vi "CalWAM-Prod(BETA).vi"(11 "error in (no error)":errorcluster) -> (4 "reference out":refnum<vi>, 15 "error out":errorcluster)   [LabVIEW 2018]
uses:
  <vilib>/Utility/file.llb/Write Delimited Spreadsheet (string).vi
  <vilib>/Utility/file.llb/Write Delimited Spreadsheet (DBL).vi
  Instruments/Keysight U2022 Power Sensor/Agilent U2000 Series/Agilent U2000 Series.lvlib
  Instruments/Agilent PSG MXG Series/Agilent PSG MXG Series.lvlib
panel:
  in  "gantry_Required(t)":bool=TRUE
  in  "Gantry":refnum<visa-resource-name>="COM5"
  in  "Path":u16(ring)=3 items=["INPUT", "FLATTEN", "OUTPUT"]
  out "IsPSA?(t)":bool
  out "SA_Offset":dbl=-100.433
  out "sg_flat_temp":path=path "C:/Users/ThomasWattson/AppData/Local/Temp/lvtemporary_990258.cal"
  out "in_cal_temp":path=path "C:/Users/ThomasWattson/AppData/Local/Temp/lvtemporary_29106.cal"
  out "out_cal_tmp":path=path "C:/Users/ThomasWattson/AppData/Local/Temp/lvtemporary_754512.cal"
  out "in_cal_file":path=path "C:/RageATE/Automated Tests/Tetra WAM/PRODUCTION/Test Benches/WAM_PROD_TEST-2/Calibration Files/WAM_PROD_TEST-2_INPUT_072523-1034.csv"
  out "date/time string":string="072523-1034"
  out "TestBench_ID":string="WAM_PROD_TEST-2"
  out "Cancel_@_Inst":bool
  in  "Tab Control":enum32{"CAL", "INST"}(tab)
  out "Switch_Present?(t)":bool=TRUE
  out "PM_Present?(t)":bool=TRUE
  out "VNA_Present?(t)":bool=TRUE
  out "MXG_Present?(t)":bool=TRUE
  out "MXA_Present?(t)":bool=TRUE
  in  "stop":bool
  out "Progress":u8(slide) caption="Input Cal 100% Complete" scale=0.0..100.0
  out "Status":string="Starting:  CalWAM-Prod(BETA).vi\rChecking Equipment..."
  out "Spec An":dbl[](array[numeric])=[11000.0, -100.433]
  out "Power Meter":dbl[](array[numeric])=[10000.0, -41.4955603]
  in  "USB Power Meter":refnum<visa-resource-name>="USB0::0x2A8D::0x7F18::MY58240013::INSTR"
  in  "VNA":refnum<visa-resource-name>="TCPIP0::169.254.70.180::inst0::INSTR"
  in  "SA":refnum<visa-resource-name>="TCPIP0::169.254.70.120::inst0::INSTR"
  in  "Sig Gen":refnum<visa-resource-name>="TCPIP0::169.254.70.100::inst0::INSTR"
  in  "PM_AVGs":i16=4
  in  "SA_AVGs":i16=8
  in  "Switch":refnum<visa-resource-name>="GPIB0::29::INSTR"
  in  "MXA_Required(t)":bool=TRUE
  in  "Preset_MXA(t)":bool=TRUE
  in  "Preset_MXG(t)":bool=TRUE
  in  "Preset_PNA(t)":bool=TRUE
  in  "Preset_PM(t)":bool=TRUE
  in  "MXG_Required(t)":bool=TRUE
  in  "PNA_Required(t)":bool=TRUE
  in  "PM_Required(t)":bool=TRUE
  in  "Switch_Required(t)":bool=TRUE
  in  "Preset_Switch(t)":bool=TRUE
  in  "Use Flatten File(t)":bool
  out "OK(t)":bool=TRUE caption="OK"
  in  "zero/cal":bool=TRUE
  in  "Span(MHz)":dbl=0.1 format="%#_13g"
  in  "RBW(Hz)":string="3000"
  in  "SA_REF_LVL (dBm)":string="0"
  in  "Input Power to Set (dBm)":dbl
  in  "SG1 delay(ms)":i64=20 caption="Delay Time (s)"
  in  "Freq Control":T1={"Start Freq (MHz)"=9000.0, "Stop Freq (MHz)"=40000.0, " Step (MHz)"=50.0}
  in  "Select AutoCal(T)":bool=TRUE
  out "GantryNOTOk?(t)":bool
  out "sg_flat_file":path=path "C:/RageATE/Automated Tests/Tetra WAM/PRODUCTION/Test Benches/WAM_PROD_TEST-2/Calibration Files/WAM_PROD_TEST-2_SG-FLAT_072523-1034.csv"
  in  "Browse for Flatness File(t)":bool
  in  "Flatness File(browse)":path
  in  "ATT":dbl format="%#_13g"
  in  "Internal Preamp (0: Off)":i32(ring)=2 items=["Off", "Low Band", "Full Range"]
  in  "Output Power to Set (dBm)":dbl=-50.0
  in  "Flatten Power to Set (dBm)":dbl
  in  "base path":path=path "C:/RageATE-Tetra/Automated Tests/Tetra WAM/PRODUCTION/Test Benches"
  out "Path_out(str)":string="OUTPUT"
  out "Flat_Cable_Data":dbl[][](array[numeric])
  out "out_cal_file":path=path "C:/RageATE/Automated Tests/Tetra WAM/PRODUCTION/Test Benches/WAM_PROD_TEST-2/Calibration Files/WAM_PROD_TEST-2_OUTPUT_072523-1034.csv"
  out "Freq_MHz (ary)":dbl[](array[numeric])=[9000.0, 9500.0, 10000.0]
  out "Ary size(s)":i32=3
  # "Set Cal Freq"
  # "FREQ (MHz)      dBm"
  # "FREQ (MHz)      dBm"
  # "PWR Meter Result"
  # "Spec An Result"
  # "INSTRUMENT Settings"
  # "Stimulus"
  # "SPEC AN"
  # "Power Meter"
  # "# of Averages ( PWR Meter and Spec An)"
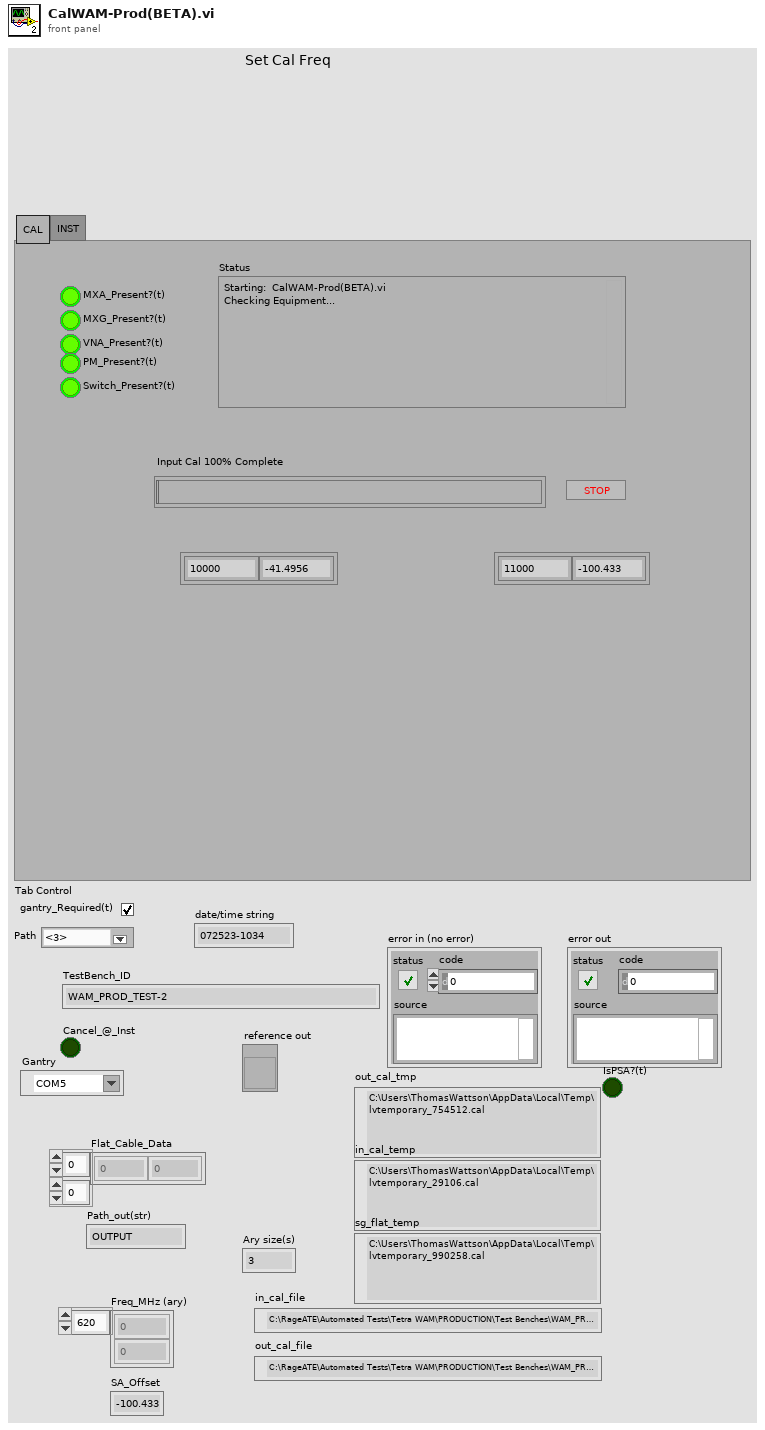
[diagram p1: front panel]
types:
  T1 = cluster{"Start Freq (MHz)":dbl, "Stop Freq (MHz)":dbl, " Step (MHz)":dbl}
  T2 = enum32{"Invalid", "Standard", "Closed", "Hidden", "Minimized", "Maximized"}
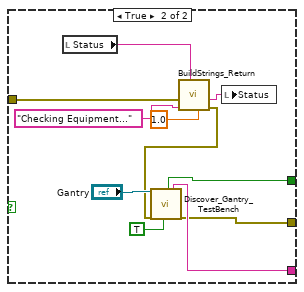
[diagram p2: hidden frame]
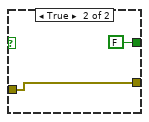
[diagram p3: hidden frame]
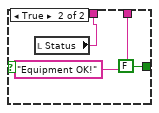
[diagram p4: hidden frame]
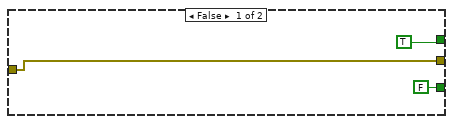
[diagram p5: hidden frame]
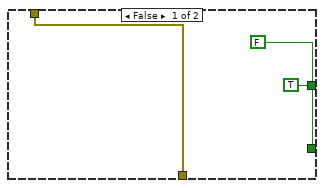
[diagram p7: hidden frame]
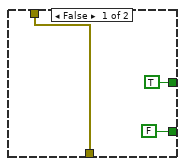
[diagram p9: hidden frame]
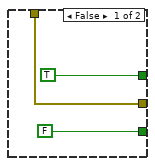
[diagram p11: hidden frame]
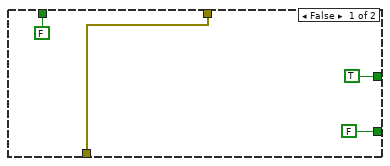
[diagram p13: hidden frame]
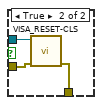
[diagram p14: hidden frame]
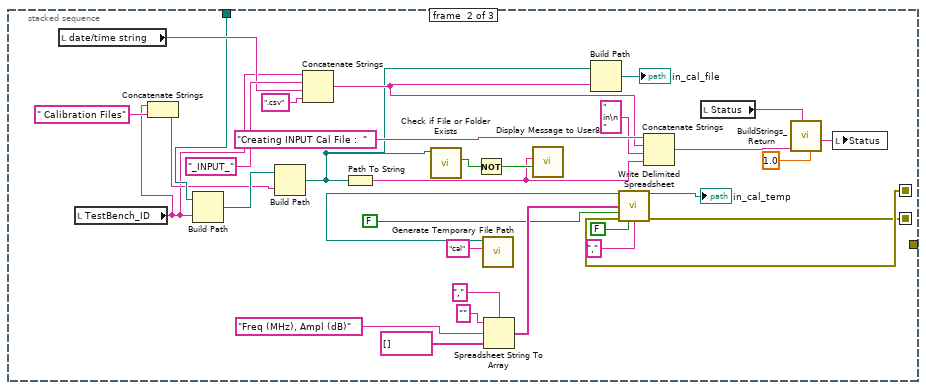
[diagram p15: hidden frame]
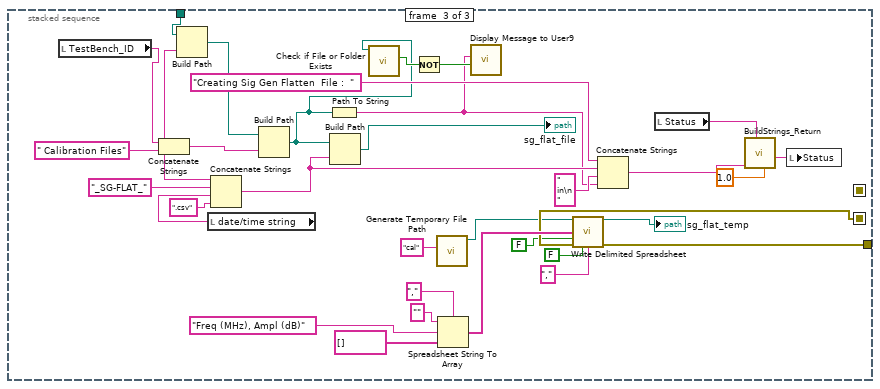
[diagram p16: hidden frame]
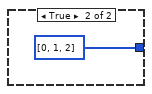
[diagram p18: hidden frame]
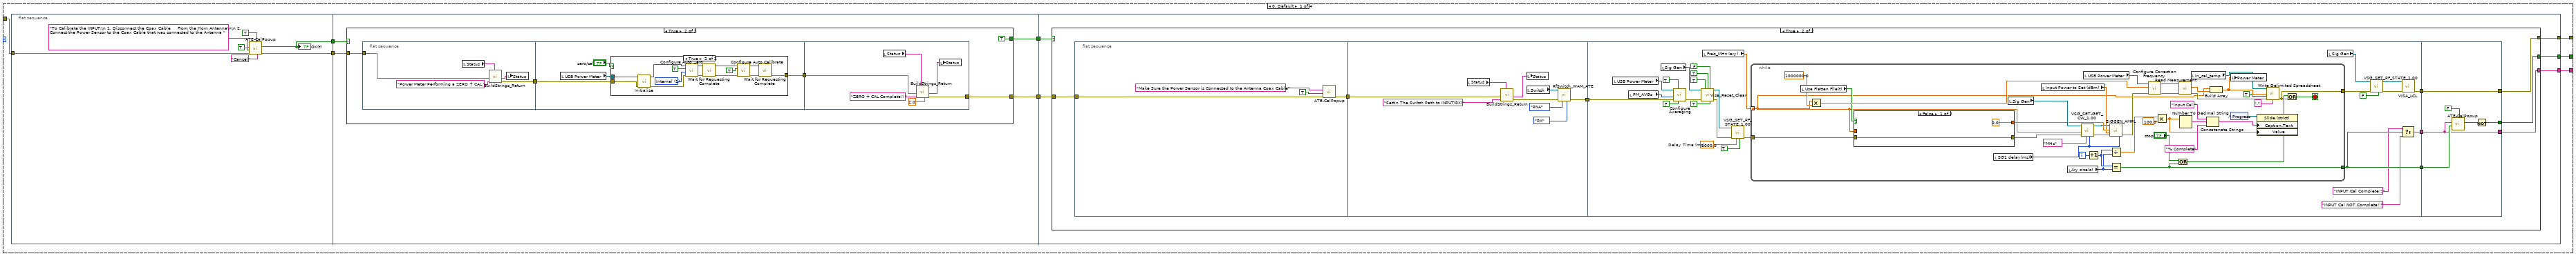
[diagram p19: hidden frame]
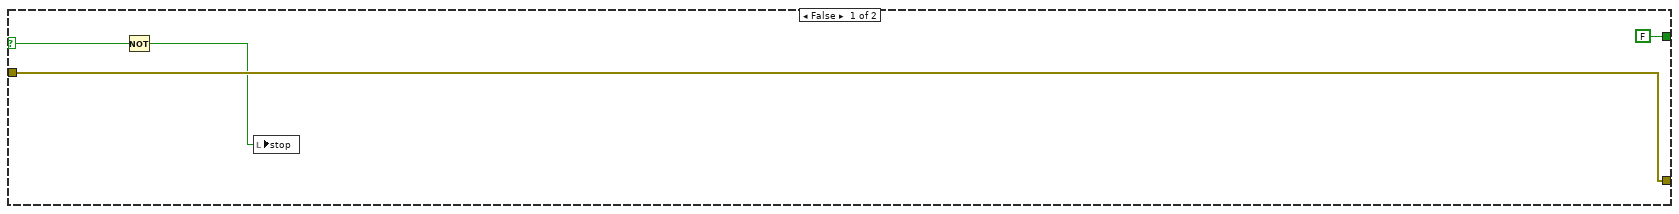
[diagram p20: hidden frame]
diagram:
  n1 = flat-sequence {
    tunnel: "error in (no error)" -> [w24]
    tunnel: [w24] -> w2
    tunnel: w2 -> [w30]
    tunnel: [w29] -> w1
    tunnel: w1 -> [w75]
    tunnel: [w71] -> w6
    tunnel: [w70] -> w5
    tunnel: [w191] -> w7
    tunnel: w6 -> [_]
    tunnel: w5 -> [w191]
    tunnel: [w201] -> w8
    tunnel: w7 -> [w202]
    tunnel: w8 -> [w312]
    tunnel: [w310] -> w3
    tunnel: [w823] -> w4
    tunnel: w3 -> [w824]
    tunnel: w4 -> [w856]
    frame #0 {
      w10 = FALSE ("MXG_Present?(t)")
      n2 = control-ref of="Status"() -> (w27:refnum<vi>)
      n3 = local write "stop"(FALSE ("stop")) -> ()
      n4 = property on="Progress" class="Slide (strict)"("Scale.Maximum"=100.0 ("Scale.Range:Maximum"), "Scale.Minimum"=0.0 ("Scale.Range:Minimum")) -> ()  [unwired: 2 in, 2 out]
      n5 = property class="Str"(reference=w27, "Value"="") -> (error out=w22:errorcluster)  [unwired: 1 in, 1 out]
      n6 = control-ref of="Progress"() -> (w19:refnum<vi>)
      n7 = invoke class="VI" method="FP.Open"("Activate"=TRUE ("Activate?"), "State"=T2."Standard") -> ()  [unwired: 3 in, 5 out]
      n8 = local write "Switch_Present?(t)"(w10) -> ()
      n9 = local write "GantryNOTOk?(t)"(w10) -> ()
      n10 = local write "IsPSA?(t)"(w10) -> ()
      n11 = local write "MXA_Present?(t)"(w10) -> ()
      n12 = local write "VNA_Present?(t)"(w10) -> ()
      n13 = property class="Slide (strict)"(reference=w19, "Caption.Text"="Resetting..." ("Label.Text")) -> ()  [unwired: 1 in, 2 out]
      n14 = control-ref of="This VI"() -> (w28:refnum<vi>)
      n15 = local write "MXG_Present?(t)"(w10) -> ()
      n16 = local write "Cancel_@_Inst"(w10) -> ()
      n17 = property on="Tab Control" class="TabCtl (strict)"("Value"=enum32{"CAL", "INST"}."CAL" ("Tab Control")) -> ()  [unwired: 2 in, 2 out]
      n18 = property class="VI"(reference=w28, error in=w22) -> (reference out=→"reference out":refnum<vi>, "Name"=w25:string)  [unwired: 1 out]
      n19 = Concatenate Strings("Starting:  " ("Status"), w25) -> (→"Status":string)
      "Progress" <- u8 0 ("Progress")
    }
    frame #1 {
      n20 = flat-sequence {
        tunnel: w30 -> [w33]
        tunnel: [w32] -> w29
        frame #0 {
          n21 = case shown="False" "gantry_Required(t)" {
            tunnel: [w38 w50] -> w37
            tunnel: [w39 w48] -> w36
            tunnel: w33 -> [w40 w43]
            tunnel: [w40 w41] -> w31
            frame False {
              n22 = call "SelectTester-PopUp.vi"() -> ("Input"=w39:string, "OK"=w38:bool)  [unwired: 17 in, 1 out]
            }
            frame True {
              n23 = local read "Status"() -> (w47:string)
              n24 = call "BuildStrings_Return.vi"("seconds to wait"=1.0, "Input String"=w47, "New String"="Checking Equipment...", "error in (no error)"=w43) -> ("error out"=w42:errorcluster, "concatenated string"=w46:string)  [unwired: 5 in, 1 out]
              n25 = call "Discover_Gantry_TestBench.vi"("Session In"="Gantry", "error in"=w42, "Close Session(t)"=TRUE) -> ("Gantry Present(t)"=w50:bool, "TestBench_ID"=w48:string, "error out"=w41:errorcluster)  [unwired: 8 in, 6 out]
              n26 = local write "Status"(w46) -> ()
            }
          }
          "TestBench_ID" <- w36
          n27 = case shown="False" w37 {
            tunnel: [w52 FALSE ("OK")] -> w35
            tunnel: [w53 w54] -> w32
            tunnel: w31 -> [w53 w54]
            frame False {
              n28 = call "Display Message to User2"() -> ("OK"=w52:bool)  [unwired: 10 in, 1 out]
            }
            frame True {
            }
          }
          "GantryNOTOk?(t)" <- w35
        }
      }
    }
    frame #2 {
      n29 = local read "Status"() -> (w62:string)
      n30 = call "BuildStrings_Return.vi"("seconds to wait"=1.0, "Input String"=w62, "New String"="Checking Equipment...", "error in (no error)"=w75) -> ("error out"=w59:errorcluster, "concatenated string"=w73:string)  [unwired: 5 in, 1 out]
      n31 = local write "Status"(w73) -> ()
      n32 = case shown="True" "Switch_Required(t)" {
        selector: "Switch_Required(t)" -> [_ w106]
        tunnel: [FALSE ("Success?(t)") w107] -> w84
        tunnel: [TRUE w105] -> w82
        tunnel: [w99 w104] -> w61
        tunnel: w59 -> [w99 w103]
        frame False {
        }
        frame True {
          n33 = call "Discover_Switch.vi"("error in"=w103, "Session In"="Switch") -> ("error out"=w102:errorcluster, "Success?(t)"=w107:bool, "Session Out"=w109:refnum<visa-resource-name>)  [unwired: 7 in]
          n34 = And(x="Preset_Switch(t)", y=w107) -> (x .and. y?=w111:bool)
          n35 = case shown="True" w111 {
            tunnel: w109 -> [_ w115]
            tunnel: [w112 w114] -> w104
            tunnel: w102 -> [w112 w113]
            frame False {
            }
            frame True {
              n36 = call "VISA_RESET-CLS.vi"("error in"=w113, "Session In"=w115) -> ("error out"=w114:errorcluster)  [unwired: 8 in, 1 out]
            }
          }
          n37 = And(x=w106, y=w107) -> (x .and. y?=w105:bool)
        }
      }
      "Switch_Present?(t)" <- w84
      n38 = case shown="True" "MXA_Required(t)" {
        selector: "MXA_Required(t)" -> [_ w181]
        tunnel: [FALSE ("Success?(t)") w182] -> w91
        tunnel: [TRUE w180] -> w80
        tunnel: [FALSE ("IsPSA?(t)") w179] -> w64
        tunnel: w61 -> [w172 w176]
        tunnel: [w172 w178] -> w60
        frame False {
        }
        frame True {
          n39 = call "Discover_MXA.vi"("error in"=w176, "Session In"="SA") -> ("error out"=w177:errorcluster, "Success?(t)"=w182:bool, "Session Out"=w183:refnum<visa-resource-name>, "IsPSA?(t)"=w179:bool)  [unwired: 5 in, 1 out]
          n40 = And(x="Preset_MXA(t)", y=w182) -> (x .and. y?=w185:bool)
          n41 = case shown="False" w185 {
            tunnel: w183 -> [_ w190]
            tunnel: [w187 w189] -> w178
            tunnel: w177 -> [w187 w188]
            frame False {
            }
            frame True {
              n42 = call "VISA_RESET-CLS.vi"("error in"=w188, "Session In"=w190) -> ("error out"=w189:errorcluster)  [unwired: 8 in, 1 out]
            }
          }
          n43 = And(x=w181, y=w182) -> (x .and. y?=w180:bool)
        }
      }
      "MXA_Present?(t)" <- w91
      "IsPSA?(t)" <- w64
      n44 = case shown="True" "PM_Required(t)" {
        tunnel: [FALSE ("Success?(t)") w123] -> w88
        tunnel: w59 -> [_ _]
        tunnel: [TRUE w121] -> w81
        tunnel: w60 -> [w116 w120]
        tunnel: [w116 w119] -> w58
        frame False {
        }
        frame True {
          n45 = call "Initialize.vi"("error in (no error)"=w120, "Reset (True)"=FALSE, "ID Query (True)"=TRUE, "VISA resource name"="USB Power Meter") -> ("error out"=w124:errorcluster, "VISA resource name out"=w126:refnum<visa-resource-name>, "Success?(t)"=w123:bool)  [unwired: 4 in, 1 out]
          n46 = And(x="Preset_PM(t)", y=w123) -> (x .and. y?=w129:bool)
          n47 = case shown="True" w129 {
            tunnel: w126 -> [_ w133]
            tunnel: w124 -> [w130 w132]
            tunnel: [w130 w131] -> w119
            frame False {
            }
            frame True {
              n48 = call "Reset.vi"("error in (no error)"=w132, "VISA resource name"=w133) -> ("error out"=w131:errorcluster)  [unwired: 8 in, 1 out]
            }
          }
          n49 = And(x="Preset_PM(t)", y=w123) -> (x .and. y?=w121:bool)
        }
      }
      "PM_Present?(t)" <- w88
      n50 = case shown="True" "PNA_Required(t)" {
        selector: "PNA_Required(t)" -> [_ w141]
        tunnel: [FALSE ("Success?(t)") w142] -> w89
        tunnel: [TRUE w140] -> w79
        tunnel: w58 -> [w134 w137]
        tunnel: [w134 w139] -> w57
        frame False {
        }
        frame True {
          n51 = call "Discover_PNA.vi"("error in"=w137, "Session In"="VNA") -> ("error out"=w138:errorcluster, "Success?(t)"=w142:bool, "Session Out"=w143:refnum<visa-resource-name>)  [unwired: 7 in]
          n52 = And(x="Preset_PNA(t)", y=w142) -> (x .and. y?=w145:bool)
          n53 = case shown="True" w145 {
            tunnel: w143 -> [_ w150]
            tunnel: [w147 w149] -> w139
            tunnel: w138 -> [w147 w148]
            frame False {
            }
            frame True {
              n54 = call "VISA_RESET-CLS.vi"("error in"=w148, "Session In"=w150) -> ("error out"=w149:errorcluster)  [unwired: 8 in, 1 out]
            }
          }
          n55 = And(x=w141, y=w142) -> (x .and. y?=w140:bool)
        }
      }
      "VNA_Present?(t)" <- w89
      n56 = case shown="True" "MXG_Required(t)" {
        selector: "MXG_Required(t)" -> [_ w158]
        tunnel: [FALSE ("Success?(t)") w159] -> w90
        tunnel: [TRUE w157] -> w78
        tunnel: w57 -> [w151 w155]
        tunnel: [w151 w156] -> w56
        frame False {
        }
        frame True {
          n57 = call "Discover_MXG.vi"("error in"=w155, "Session In"="Sig Gen") -> ("error out"=w154:errorcluster, "Success?(t)"=w159:bool, "Session Out"=w162:refnum<visa-resource-name>)  [unwired: 7 in]
          n58 = And(x=w159, y="Preset_MXG(t)") -> (x .and. y?=w161:bool)
          n59 = case shown="True" w161 {
            tunnel: w162 -> [_ w171]
            tunnel: [w164 w166] -> w156
            tunnel: w154 -> [w164 w165]
            frame False {
            }
            frame True {
              n60 = call "Reset.vi"("error in (no error)"=w165, "VISA resource name"=w171) -> ("error out"=w170:errorcluster, "VISA resource name out"=w169:refnum<visa-resource-name>)  [unwired: 8 in]
              n61 = call "Initialize.vi"("error in (no error)"=w170, "VISA resource name"=w169) -> ("error out"=w167:errorcluster, "VISA resource name out"=w168:refnum<visa-resource-name>)  [unwired: 8 in]
              n62 = call "Flatness_PreSet.vi"("error in"=w167, "Session In"=w168) -> ("error out"=w166:errorcluster)  [unwired: 7 in, 1 out]
            }
          }
          n63 = And(x=w158, y=w159) -> (x .and. y?=w157:bool)
        }
      }
      "MXG_Present?(t)" <- w90
      n64 = Build Array(w82, w81, w80, w79, w78) -> (w77:bool[])
      n65 = And Array Elements(Boolean array=w77) -> (logical AND=w76:bool)
      n66 = case shown="False" w76 {
        tunnel: [w95 FALSE ("OK")] -> w65
        tunnel: ["Equipment ISSUE!" ("New String") "Equipment OK!" ("New String")] -> w71
        tunnel: [w93 w96] -> w67
        frame False {
          n67 = local read "Status"() -> (w93:string)
          n68 = call "Display Message to User"() -> ("Cancel (End)"=w95:bool)  [unwired: 10 in, 1 out]
        }
        frame True {
          n69 = local read "Status"() -> (w96:string)
        }
      }
      n70 = local read "GantryNOTOk?(t)"() -> (w63:bool)
      n71 = Or(x=w63, y=w65) -> (x .or. y?=→"Cancel_@_Inst":bool)
      n72 = call "BuildStrings_Return.vi"("seconds to wait"=1.0, "Input String"=w67, "New String"=w71, "error in (no error)"=w56) -> ("error out"=w70:errorcluster, "concatenated string"=w69:string)  [unwired: 5 in, 1 out]
      n73 = local write "Status"(w69) -> ()
    }
    frame #3 {
      n74 = call "Ramp-Step.vi"("Controls"="Freq Control") -> ("Ary size(s)"=→"Ary size(s)":i32, "Freq (ary)"=→"Freq_MHz (ary)":dbl[])  [unwired: 11 in, 2 out]
      n75 = Get Date/Time In Seconds() -> (seconds since 1Jan1904=w194:timestamp)
      n76 = Format Date/Time String(time format string (%c)="%m%d%y-%H%M", seconds (now)=w194) -> (date/time string=→"date/time string":string)  [unwired: 1 in]
      "Power Meter" <- dbl[] []
    }
    frame #4 {
      n77 = local read "Cancel_@_Inst"() -> (w200:bool)
      n78 = case shown="False" w200 {
        tunnel: w202 -> [w205 w306]
        tunnel: [w204 w306] -> w201
        tunnel: "base path" -> [w203 _]
        frame False {
          n79 = stacked-sequence "Create The Files" {
            seq-local: [w228 _ _] -> [_ w262 _]
            seq-local: [_ w261 _] -> [_ _ w295]
            tunnel: w205 -> [w239 _ _]
            tunnel: [_ _ w294] -> w204
            tunnel: w203 -> [w212 w246 w279]
            frame #0 {
              n80 = call <vilib>:"Generate Temporary File Path.vi"("Temporary File Extension (tmp)"="cal") -> ("Unique Temporary File Path"=w215:path)  [unwired: 9 in, 1 out]
              n81 = Spreadsheet String To Array(delimiter (Tab)=",", format string="", spreadsheet string="Freq (MHz), Ampl (dB)" ("delimiter (\\t)"), array type (2D Dbl)=string[] []) -> (array=w234:string[])
              n82 = local read "TestBench_ID"() -> (w210:string)
              n83 = call-poly <vilib>:"Write Delimited Spreadsheet.vi"("file path (dialog if empty)"=w215, "1D data"=w234, "append to file? (new file:F)"=FALSE, "error in (no error)"=w239, "transpose? (no:F)"=FALSE, "delimiter (\\t)"="," ("delimiter (\\t)")) -> ("new file path (Not A Path if cancelled)"=→"out_cal_tmp":path, "error out"=w228:errorcluster)  [unwired: 8 in]
              n84 = local read "date/time string"() -> (w230:string)
              n85 = Concatenate Strings(w210, " Calibration Files" ("name or relative path")) -> (w211:string)
              n86 = Build Path(base path=w212, name or relative path=w210) -> (appended path=w226:path)
              n87 = Concatenate Strings(w210, "_OUTPUT_" ("string"), w230, ".csv" ("name or relative path")) -> (w223:string)
              n88 = Build Path(base path=w226, name or relative path=w211) -> (appended path=w207:path)
              n89 = call <vilib>:"Check if File or Folder Exists.vi"("path"=w207) -> ("file or folder exists?"=w209:bool)  [unwired: 8 in, 2 out]
              n90 = Path To String(path=w207) -> (string=w206:string)
              n91 = Not(x=w209) -> (.not. x?=w208:bool)
              n92 = Path To String(path=w207) -> (string=w221:string)
              n93 = call "Display Message to User7"("Enable"=w208, "Message"=w206) -> ()  [unwired: 8 in, 2 out]
              n94 = Concatenate Strings("Creating OUTPUT Cal File :  " ("New String"), w223, " in\n " ("string"), w221) -> (w224:string)
              n95 = Build Path(base path=w207, name or relative path=w223) -> (appended path=→"out_cal_file":path)
              n96 = local read "Status"() -> (w225:string)
              n97 = call "BuildStrings_Return.vi"("seconds to wait"=1.0, "Input String"=w225, "New String"=w224) -> ("concatenated string"=w220:string)  [unwired: 6 in, 2 out]
              n98 = local write "Status"(w220) -> ()
            }
            frame #1 {
              n99 = local read "date/time string"() -> (w264:string)
              n100 = local read "TestBench_ID"() -> (w244:string)
              n101 = Concatenate Strings(w244, " Calibration Files" ("name or relative path")) -> (w245:string)
              n102 = Build Path(base path=w246, name or relative path=w244) -> (appended path=w259:path)
              n103 = Build Path(base path=w259, name or relative path=w245) -> (appended path=w240:path)
              n104 = Concatenate Strings(w244, "_INPUT_" ("string"), w264, ".csv" ("name or relative path")) -> (w252:string)
              n105 = Path To String(path=w240) -> (string=w241:string)
              n106 = call <vilib>:"Check if File or Folder Exists.vi"("path"=w240) -> ("file or folder exists?"=w243:bool)  [unwired: 8 in, 2 out]
              n107 = Not(x=w243) -> (.not. x?=w242:bool)
              n108 = call <vilib>:"Generate Temporary File Path.vi"("Temporary File Extension (tmp)"="cal") -> ("Unique Temporary File Path"=w249:path)  [unwired: 9 in, 1 out]
              n109 = Spreadsheet String To Array(delimiter (Tab)=",", format string="", spreadsheet string="Freq (MHz), Ampl (dB)" ("delimiter (\\t)"), array type (2D Dbl)=string[] []) -> (array=w268:string[])
              n110 = call "Display Message to User8"("Enable"=w242, "Message"=w241) -> ()  [unwired: 8 in, 2 out]
              n111 = Build Path(base path=w240, name or relative path=w252) -> (appended path=→"in_cal_file":path)
              n112 = call-poly <vilib>:"Write Delimited Spreadsheet.vi"("file path (dialog if empty)"=w249, "1D data"=w268, "append to file? (new file:F)"=FALSE, "error in (no error)"=w262, "transpose? (no:F)"=FALSE, "delimiter (\\t)"="," ("delimiter (\\t)")) -> ("new file path (Not A Path if cancelled)"=→"in_cal_temp":path, "error out"=w261:errorcluster)  [unwired: 8 in]
              n113 = Concatenate Strings("Creating INPUT Cal File :  " ("New String"), w252, " in\n " ("string"), w241) -> (w257:string)
              n114 = local read "Status"() -> (w258:string)
              n115 = call "BuildStrings_Return.vi"("seconds to wait"=1.0, "Input String"=w258, "New String"=w257) -> ("concatenated string"=w256:string)  [unwired: 6 in, 2 out]
              n116 = local write "Status"(w256) -> ()
            }
            frame #2 {
              n117 = local read "TestBench_ID"() -> (w277:string)
              n118 = Concatenate Strings(w277, " Calibration Files" ("name or relative path")) -> (w278:string)
              n119 = Build Path(base path=w279, name or relative path=w277) -> (appended path=w292:path)
              n120 = local read "date/time string"() -> (w304:string)
              n121 = Concatenate Strings(w277, "_SG-FLAT_" ("string"), w304, ".csv" ("name or relative path")) -> (w284:string)
              n122 = Build Path(base path=w292, name or relative path=w278) -> (appended path=w273:path)
              n123 = Path To String(path=w273) -> (string=w274:string)
              n124 = Build Path(base path=w273, name or relative path=w284) -> (appended path=→"sg_flat_file":path)
              n125 = call <vilib>:"Check if File or Folder Exists.vi"("path"=w273) -> ("file or folder exists?"=w276:bool)  [unwired: 8 in, 2 out]
              n126 = Not(x=w276) -> (.not. x?=w275:bool)
              n127 = call <vilib>:"Generate Temporary File Path.vi"("Temporary File Extension (tmp)"="cal") -> ("Unique Temporary File Path"=w281:path)  [unwired: 9 in, 1 out]
              n128 = Spreadsheet String To Array(delimiter (Tab)=",", format string="", spreadsheet string="Freq (MHz), Ampl (dB)" ("delimiter (\\t)"), array type (2D Dbl)=string[] []) -> (array=w305:string[])
              n129 = call "Display Message to User9"("Enable"=w275, "Message"=w274) -> ()  [unwired: 8 in, 2 out]
              n130 = call-poly <vilib>:"Write Delimited Spreadsheet.vi"("file path (dialog if empty)"=w281, "1D data"=w305, "append to file? (new file:F)"=FALSE, "error in (no error)"=w295, "transpose? (no:F)"=FALSE, "delimiter (\\t)"="," ("delimiter (\\t)")) -> ("new file path (Not A Path if cancelled)"=→"sg_flat_temp":path, "error out"=w294:errorcluster)  [unwired: 8 in]
              n131 = Concatenate Strings("Creating Sig Gen Flatten  File :  " ("New String"), w284, " in\n " ("string"), w274) -> (w289:string)
              n132 = local read "Status"() -> (w290:string)
              n133 = call "BuildStrings_Return.vi"("seconds to wait"=1.0, "Input String"=w290, "New String"=w289) -> ("concatenated string"=w288:string)  [unwired: 6 in, 2 out]
              n134 = local write "Status"(w288) -> ()
            }
          }
        }
        frame True {
        }
      }
    }
    frame #5 {
      n135 = local read "Cancel_@_Inst"() -> (w307:bool)
      n136 = case shown="False" w307 {
        tunnel: [w319 w813] -> w313
        tunnel: w312 -> [w318 w813]
        tunnel: [w317 "Calibration Cancelled!!" ("Message")] -> w311
        tunnel: [w316 FALSE] -> w309
        frame False {
          n137 = case shown="False" "Select AutoCal(T)" {
            tunnel: [w321 u16[] [0, 1, 2] ("f")] -> w314
            frame False {
              n138 = call "PathSelectPopUp.vi"("Enable"=TRUE) -> ("PATH"=w320:u16)  [unwired: 16 in, 2 out]
              n139 = local write "Path"(w320) -> ()
              n140 = Build Array(w320) -> (w321:u16[])
            }
            frame True {
            }
          }
          n141 = while {
            tunnel: w314 -> [w327] mode=indexing
            shift-right: [w331] -> w319
            shift-left: w318 -> [w330]
            tunnel: [w326] -> w316
            tunnel: [w328] -> w317
            stop <- w326 stop-if-true
            n142 = case shown="2" w327 {
              selector: w327 -> [_ _ w672 _]
              tunnel: [w336 w503 w666 w810] -> w331
              tunnel: w330 -> [w338 w505 w668 w810]
              tunnel: [w335 w502 w661 TRUE ("OK")] -> w329
              tunnel: [w332 w501 w660 "SKipped" ("Message")] -> w328
              frame 0, Default {
                n143 = flat-sequence {
                  tunnel: [w344] -> w339
                  tunnel: w338 -> [w343]
                  tunnel: [w342] -> w334
                  tunnel: w339 -> [w349]
                  tunnel: [w350] -> w337
                  tunnel: w334 -> [w348]
                  tunnel: [w347] -> w333
                  tunnel: w337 -> [w395]
                  tunnel: [w396] -> w336
                  tunnel: [w394] -> w335
                  tunnel: w333 -> [w393]
                  tunnel: [w392] -> w332
                  frame #0 {
                    n144 = call "ATE-CalPopup.vi"("Second Button Name"="Cancel", "Show 'Cancel' Button"=TRUE, "error in (no error)"=w343, "Enable"=TRUE, "Message"="To Calibrate the INPUT:\n 1. Disconnect the Coax Cable     From the Horn Antenna\n\n 2.Connect the Power Sensor to the Coax Cable that was connected to the Antenna ") -> ("error out"=w344:errorcluster, "OK"=w342:bool)  [unwired: 5 in]
                    "OK(t)" <- w342
                  }
                  frame #1 {
                    n145 = case shown="True" w348 {
                      selector: w348 -> [w352 _]
                      tunnel: [w354 w357] -> w350
                      tunnel: w349 -> [w354 w356]
                      tunnel: [FALSE TRUE] -> w347
                      frame False {
                        n146 = Not(x=w352) -> (.not. x?=w351:bool)
                        n147 = local write "stop"(w351) -> ()
                      }
                      frame True {
                        n148 = flat-sequence {
                          tunnel: w356 -> [w361]
                          tunnel: [w360] -> w359
                          tunnel: w359 -> [w365]
                          tunnel: [w366] -> w358
                          tunnel: [w388] -> w357
                          tunnel: w358 -> [w389]
                          frame #0 {
                            n149 = local read "Status"() -> (w364:string)
                            n150 = call "BuildStrings_Return.vi"("Input String"=w364, "New String"="Power Meter Performing a ZERO + CAL ", "error in (no error)"=w361) -> ("error out"=w360:errorcluster, "concatenated string"=w363:string)  [unwired: 6 in, 1 out]
                            n151 = local write "Status"(w363) -> ()
                          }
                          frame #1 {
                            n152 = local read "USB Power Meter"() -> (w367:refnum<visa-resource-name>)
                            n153 = case shown="True" "zero/cal" {
                              tunnel: w367 -> [w370 w383]
                              tunnel: w365 -> [w371 w381]
                              tunnel: [w369 w378] -> w366
                              frame False {
                                n154 = call "Initialize.vi"("error in (no error)"=w371, "VISA resource name"=w370) -> ("error out"=w369:errorcluster)  [unwired: 6 in, 3 out]
                              }
                              frame True {
                                w385 = 1 items=["External", "Internal"] ("Zero Type (0: External)")
                                n155 = call "Initialize.vi"("error in (no error)"=w381, "VISA resource name"=w383) -> ("error out"=w382:errorcluster, "VISA resource name out"=w384:refnum<visa-resource-name>)  [unwired: 6 in, 2 out]
                                n156 = call "Configure Auto Zero.vi"("error in (no error)"=w382, "Zero Type (0: External)"=w385, "Auto Zero (T: Enable)"=TRUE, "VISA resource name"=w384) -> ("error out"=w373:errorcluster, "VISA resource name out"=w374:refnum<visa-resource-name>)  [unwired: 6 in]
                                n157 = call "Wait for Requesting Complete.vi"("error in (no error)"=w373, "VISA resource name"=w374) -> ("error out"=w372:errorcluster, "VISA resource name out"=w375:refnum<visa-resource-name>)  [unwired: 8 in]
                                n158 = call "Configure Auto Calibrate.vi"("error in (no error)"=w372, "Auto Calibrate (T: Enable)"=TRUE, "VISA resource name"=w375) -> ("error out"=w377:errorcluster, "VISA resource name out"=w376:refnum<visa-resource-name>)  [unwired: 7 in]
                                n159 = call "Wait for Requesting Complete.vi"("error in (no error)"=w377, "VISA resource name"=w376) -> ("error out"=w378:errorcluster)  [unwired: 8 in, 1 out]
                              }
                            }
                          }
                          frame #2 {
                            n160 = local read "Status"() -> (w387:string)
                            n161 = call "BuildStrings_Return.vi"("seconds to wait"=2.0, "Input String"=w387, "New String"="ZERO + CAL Complete!! ", "error in (no error)"=w389) -> ("error out"=w388:errorcluster, "concatenated string"=w390:string)  [unwired: 5 in, 1 out]
                            n162 = local write "Status"(w390) -> ()
                          }
                        }
                      }
                    }
                  }
                  frame #2 {
                    n163 = case shown="True" w393 {
                      tunnel: [w398 w403] -> w396
                      tunnel: w395 -> [w398 w402]
                      tunnel: [TRUE w401] -> w394
                      tunnel: ["Calibration Cancelled!!!" ("Message") w400] -> w392
                      frame False {
                      }
                      frame True {
                        n164 = flat-sequence {
                          tunnel: w402 -> [w411]
                          tunnel: [w410] -> w408
                          tunnel: w408 -> [w417]
                          tunnel: [w416] -> w407
                          tunnel: w407 -> [w447]
                          tunnel: [w448] -> w406
                          tunnel: [w446] -> w405
                          tunnel: [w445] -> w404
                          tunnel: [w500] -> w403
                          tunnel: w406 -> [w500]
                          tunnel: w405 -> [w499]
                          tunnel: w404 -> [w496]
                          tunnel: [w497] -> w401
                          tunnel: [w496] -> w400
                          frame #0 {
                            n165 = call "ATE-CalPopup.vi"("error in (no error)"=w411, "Enable"=TRUE, "Message"="Make Sure the Power Sensor is Connected to the Antenna Coax Cable") -> ("error out"=w410:errorcluster)  [unwired: 7 in, 1 out]
                          }
                          frame #1 {
                            n166 = local read "Status"() -> (w420:string)
                            n167 = call "BuildStrings_Return.vi"("Input String"=w420, "New String"="Settin The Switch Path to INPUT(RX)", "error in (no error)"=w417) -> ("error out"=w415:errorcluster, "concatenated string"=w419:string)  [unwired: 6 in, 1 out]
                            n168 = local write "Status"(w419) -> ()
                            n169 = local read "Switch"() -> (w421:refnum<visa-resource-name>)
                            n170 = call "RfSwitch_WAM_ATE.vi"("VISA_IN"=w421, "error in"=w415, "Source"=enum16{"RFSM", "PNA"}."PNA", "T/R"=enum16{"TX", "RX"}."RX") -> ("error out"=w416:errorcluster)  [unwired: 10 in, 1 out]
                          }
                          frame #2 {
                            w430 = 1000.0  # Delay Time (ms)
                            n171 = local read "USB Power Meter"() -> (w428:refnum<visa-resource-name>)
                            n172 = local read "PM_AVGs"() -> (w427:i16)
                            n173 = local read "Sig Gen"() -> (w437:refnum<visa-resource-name>)
                            n174 = call "Configure Averaging.vi"("Auto Averaging (T: Enable)"=FALSE, "Enable Averaging (T: Enable)"=TRUE, "error in (no error)"=w447, "Averaging Count (4)"=w427, "VISA resource name"=w428) -> ("error out"=w429:errorcluster)  [unwired: 5 in, 1 out]
                            n175 = call "Visa_Reset_Clear.vi"("VISA resource name"=w437, "Send *CLS"=TRUE, "Restore Defaults"=TRUE, "Close VISA session"=FALSE, "error in (no error)"=w429, "Send *RST"=TRUE) -> ("VISA resource name Out"=w436:refnum<visa-resource-name>, "error out"=w435:errorcluster)  [unwired: 8 in]
                            n176 = local read "Freq_MHz (ary)"() -> (w444:dbl[])
                            n177 = call "VSG_SET_RF_STATE_1.00.vi"("RF ON/OFF (OFF)"=TRUE, "Delay Time (ms)"=w430, "error in"=w435, "Session In"=w436) -> ("error out"=w443:errorcluster)  [unwired: 5 in, 2 out]
                            n178 = while {
                              tunnel: [w469] -> w425
                              tunnel: w444 -> [w459] mode=indexing
                              tunnel: w443 -> [w482]
                              tunnel: [w467] -> w446
                              i -> [w483]
                              stop <- w470 stop-if-true
                              n179 = local read "Use Flatten File(t)"() -> (w473:bool)
                              n180 = Multiply(x=w459, y=1000000.0) -> (x*y=w476:dbl)
                              n181 = case shown="False" w473 {
                                tunnel: w482 -> [w489 w493]
                                tunnel: [w489 w492] -> w466
                                tunnel: [0.0 ("Ampl Out") w491] -> w461
                                tunnel: w459 -> [_ w490]
                                frame False {
                                }
                                frame True {
                                n182 = local read "Flat_Cable_Data"() -> (w494:dbl[][])
                                n183 = call "GetCalData.vi"("Ary In"=w494, "error in (no error)"=w493, "RF Freq (MHz)"=w490) -> ("error out"=w492:errorcluster, "Ampl Out"=w491:dbl)  [unwired: 3 in, 4 out]
                                }
                              }
                              n184 = local read "SG1 delay(ms)"() -> (w481:i64)
                              n185 = local read "Sig Gen"() -> (w465:refnum<visa-resource-name>)
                              n186 = local read "Input Power to Set (dBm)"() -> (w460:dbl)
                              n187 = local read "Ary size(s)"() -> (w455:i32)
                              n188 = call "VSG_SET-GET_CW_1.00.vi"("Set Delay after (ms)"=w481, "Freq Units"="MHz", "error in"=w466, "Set Freq (MHz) num"=w459, "Session In"=w465) -> ("error out"=w463:errorcluster, "Session Out"=w464:refnum<visa-resource-name>)  [unwired: 3 in, 2 out]
                              n189 = local read "USB Power Meter"() -> (w472:refnum<visa-resource-name>)
                              n190 = Increment(x=w483) -> (x+1=w456:i32)
                              n191 = call "SIGGEN_AMPL.vi"("Session In"=w464, "OFFS_IN"=w461, "Set Power (num)"=w460, "error in"=w463, "delay after set (ms)"=w481) -> ("error out"=w462:errorcluster)  [unwired: 7 in, 3 out]
                              n192 = Divide(x=w456, y=w455) -> (x/y=w454:dbl)
                              n193 = Equal?(x=w456, y=w455) -> (x = y?=w467:bool)
                              n194 = call "Configure Correction Frequency.vi"("error in (no error)"=w462, "Frequency (5E+7 Hz)"=w476, "VISA resource name"=w472) -> ("error out"=w480:errorcluster, "VISA resource name out"=w474:refnum<visa-resource-name>)  [unwired: 7 in]
                              n195 = Multiply(x=w454, y=100.0) -> (x*y=w450:dbl)
                              n196 = Or(x="stop", y=w467) -> (x .or. y?=w486:bool)
                              n197 = call "Read Measurement.vi"("error in (no error)"=w480, "VISA resource name"=w474) -> ("error out"=w478:errorcluster, "Measurement"=w479:dbl)  [unwired: 7 in, 1 out]
                              n198 = Number To Decimal String(number=w450) -> (decimal integer string=w451:string)  [unwired: 1 in]
                              n199 = local read "in_cal_temp"() -> (w471:path)
                              n200 = Concatenate Strings("Input Cal " ("string"), w451, "% Complete" ("Label.Text")) -> (w452:string)
                              n201 = Build Array(w459, w479) -> (w477:dbl[])
                              n202 = local write "Power Meter"(w477) -> ()
                              n203 = control-ref of="Progress"() -> (w458:refnum<vi>)
                              n204 = property class="Slide (strict)"(reference=w458, "Caption.Text"=w452, "Value"=w450) -> ()  [unwired: 1 in, 2 out]
                              n205 = call-poly <vilib>:"Write Delimited Spreadsheet.vi"("file path (dialog if empty)"=w471, "1D data"=w477, "append to file? (new file:F)"=TRUE, "error in (no error)"=w478, "delimiter (\\t)"="," ("delimiter (\\t)")) -> ("error out"=w469:errorcluster)  [unwired: 9 in, 1 out]
                              n206 = Or(x=w486, y=w469) -> (x .or. y?=w470:bool)
                            }
                            n207 = local read "Sig Gen"() -> (w434:refnum<visa-resource-name>)
                            n208 = call "VSG_SET_RF_STATE_1.00.vi"("RF ON/OFF (OFF)"=FALSE, "error in"=w425, "Session In"=w434) -> ("error out"=w432:errorcluster, "Session Out"=w431:refnum<visa-resource-name>)  [unwired: 6 in, 1 out]
                            n209 = call "VISA_LCL.vi"("error in"=w432, "Session In"=w431) -> ("error out"=w448:errorcluster)  [unwired: 8 in, 1 out]
                            n210 = Select(t="INPUT Cal Complete!!!", s=w446, f="INPUT Cal NOT Complete!!!") -> (s? t:f=w445:string)
                          }
                          frame #3 {
                            n211 = call "ATE-CalPopup.vi"("Show 'Cancel' Button"=FALSE, "Enable"=w499, "Message"=w496) -> ("OK"=w498:bool)  [unwired: 7 in, 1 out]
                            n212 = Not(x=w498) -> (.not. x?=w497:bool)
                          }
                        }
                      }
                    }
                  }
                }
              }
              frame 1 {
                n213 = flat-sequence {
                  tunnel: [w508] -> w506
                  tunnel: w505 -> [w507]
                  tunnel: w506 -> [w512]
                  tunnel: [w515] -> w504
                  tunnel: w504 -> [w560]
                  tunnel: [w561] -> w503
                  tunnel: [w554] -> w502
                  tunnel: [w553] -> w501
                  frame #0 {
                    n214 = call "ATE-CalPopup.vi"("error in (no error)"=w507, "Enable"=TRUE, "Message"="To Calibrate the OUTPUT (Flatten Cal Cable Step):\n 1. Disconnect the Coax Cable  From the Horn Antenna\n2. Connect A Test Cable  suitable for 40 GHz That will Reach the Horn Antenna Cable End\na. Connect 1 End to The Signal Generators Output RF Connector\nb. Connect The Power Sensor to the other cable end") -> ("error out"=w508:errorcluster)  [unwired: 7 in, 1 out]
                  }
                  frame #1 {
                    n215 = flat-sequence {
                      tunnel: [w517] -> w514
                      tunnel: w512 -> [w516]
                      tunnel: w514 -> [w523]
                      tunnel: [w524] -> w513
                      tunnel: [w521] -> w511
                      tunnel: [w550] -> w515
                      tunnel: w513 -> [w551]
                      tunnel: w511 -> [w548]
                      frame #0 {
                        n216 = local read "Status"() -> (w520:string)
                        n217 = call "BuildStrings_Return.vi"("Input String"=w520, "New String"="Power Meter Initializing...", "error in (no error)"=w516) -> ("error out"=w517:errorcluster, "concatenated string"=w519:string)  [unwired: 6 in, 1 out]
                        n218 = local write "Status"(w519) -> ()
                      }
                      frame #1 {
                        n219 = local read "USB Power Meter"() -> (w525:refnum<visa-resource-name>)
                        n220 = case shown="False" FALSE {
                          tunnel: w525 -> [w531 w545]
                          tunnel: w523 -> [w532 w543]
                          tunnel: [w530 w540] -> w524
                          tunnel: [w526 ""] -> w521
                          frame False {
                            n221 = call "Initialize.vi"("error in (no error)"=w532, "VISA resource name"=w531) -> ("error out"=w530:errorcluster, "Success?(t)"=w527:bool)  [unwired: 6 in, 2 out]
                            n222 = Select(t="Initialization Complete!! ", s=w527, f="Initialization Error!! ") -> (s? t:f=w526:string)
                          }
                          frame True {
                            w547 = 1 items=["External", "Internal"] ("Zero Type (0: External)")
                            n223 = call "Initialize.vi"("error in (no error)"=w543, "VISA resource name"=w545) -> ("error out"=w544:errorcluster, "VISA resource name out"=w546:refnum<visa-resource-name>)  [unwired: 6 in, 2 out]
                            n224 = call "Configure Auto Zero.vi"("error in (no error)"=w544, "Zero Type (0: External)"=w547, "Auto Zero (T: Enable)"=TRUE, "VISA resource name"=w546) -> ("error out"=w535:errorcluster, "VISA resource name out"=w536:refnum<visa-resource-name>)  [unwired: 6 in]
                            n225 = call "Wait for Requesting Complete.vi"("error in (no error)"=w535, "VISA resource name"=w536) -> ("error out"=w534:errorcluster, "VISA resource name out"=w537:refnum<visa-resource-name>)  [unwired: 8 in]
                            n226 = call "Configure Auto Calibrate.vi"("error in (no error)"=w534, "Auto Calibrate (T: Enable)"=TRUE, "VISA resource name"=w537) -> ("error out"=w539:errorcluster, "VISA resource name out"=w538:refnum<visa-resource-name>)  [unwired: 7 in]
                            n227 = call "Wait for Requesting Complete.vi"("error in (no error)"=w539, "VISA resource name"=w538) -> ("error out"=w540:errorcluster)  [unwired: 8 in, 1 out]
                          }
                        }
                      }
                      frame #2 {
                        n228 = local read "Status"() -> (w549:string)
                        n229 = call "BuildStrings_Return.vi"("Input String"=w549, "New String"=w548, "error in (no error)"=w551) -> ("error out"=w550:errorcluster, "concatenated string"=w552:string)  [unwired: 6 in, 1 out]
                        n230 = local write "Status"(w552) -> ()
                      }
                    }
                  }
                  frame #2 {
                    n231 = flat-sequence {
                      tunnel: w560 -> [w564]
                      tunnel: [w563] -> w559
                      tunnel: w559 -> [w569]
                      tunnel: [w568] -> w558
                      tunnel: w558 -> [w604]
                      tunnel: [w605] -> w557
                      tunnel: [w603] -> w556
                      tunnel: [w580] -> w555
                      tunnel: [w580] -> w553
                      tunnel: [w656] -> w561
                      tunnel: w557 -> [w656]
                      tunnel: w556 -> [w655]
                      tunnel: w555 -> [w654]
                      tunnel: [w652] -> w554
                      frame #0 {
                        n232 = call "ATE-CalPopup.vi"("error in (no error)"=w564, "Enable"=TRUE, "Message"="Make Sure the Power Sensor is Connected to the Test Coax Cable End \nThat will be used to connect to the Antenna Cable  ") -> ("error out"=w563:errorcluster)  [unwired: 7 in, 1 out]
                      }
                      frame #1 {
                        n233 = local read "Status"() -> (w572:string)
                        n234 = call "BuildStrings_Return.vi"("Input String"=w572, "New String"="Skip Settin The Switch Path ", "error in (no error)"=w569) -> ("error out"=w567:errorcluster, "concatenated string"=w571:string)  [unwired: 6 in, 1 out]
                        n235 = local write "Status"(w571) -> ()
                        n236 = case shown="True" TRUE {
                          tunnel: [w573 w577] -> w568
                          tunnel: w567 -> [w573 w576]
                          frame False {
                          }
                          frame True {
                            n237 = local read "Switch"() -> (w578:refnum<visa-resource-name>)
                            n238 = call "RfSwitch_WAM_ATE.vi"("VISA_IN"=w578, "error in"=w576, "Source"=enum16{"RFSM", "PNA"}."PNA", "T/R"=enum16{"TX", "RX"}."TX") -> ("error out"=w577:errorcluster)  [unwired: 10 in, 1 out]
                          }
                        }
                      }
                      frame #2 {
                        w589 = 1000.0  # Delay Time (ms)
                        n239 = local read "USB Power Meter"() -> (w587:refnum<visa-resource-name>)
                        n240 = local read "PM_AVGs"() -> (w586:i16)
                        n241 = local read "Sig Gen"() -> (w596:refnum<visa-resource-name>)
                        n242 = call "Configure Averaging.vi"("Auto Averaging (T: Enable)"=FALSE, "Enable Averaging (T: Enable)"=TRUE, "error in (no error)"=w604, "Averaging Count (4)"=w586, "VISA resource name"=w587) -> ("error out"=w588:errorcluster)  [unwired: 5 in, 1 out]
                        n243 = call "Visa_Reset_Clear.vi"("VISA resource name"=w596, "Send *CLS"=TRUE, "Restore Defaults"=TRUE, "Close VISA session"=FALSE, "error in (no error)"=w588, "Send *RST"=TRUE) -> ("VISA resource name Out"=w595:refnum<visa-resource-name>, "error out"=w594:errorcluster)  [unwired: 8 in]
                        n244 = local read "Freq_MHz (ary)"() -> (w579:dbl[])
                        n245 = call "VSG_SET_RF_STATE_1.00.vi"("RF ON/OFF (OFF)"=TRUE, "Delay Time (ms)"=w589, "error in"=w594, "Session In"=w595) -> ("error out"=w602:errorcluster)  [unwired: 5 in, 2 out]
                        n246 = while {
                          tunnel: [w624] -> w584
                          tunnel: w579 -> [w634] mode=indexing
                          tunnel: w602 -> [w640]
                          tunnel: [w622] -> w603
                          i -> [w641]
                          stop <- w625 stop-if-true
                          n247 = local read "Use Flatten File(t)"() -> (w628:bool)
                          n248 = Multiply(x=w634, y=1000000.0) -> (x*y=w631:dbl)
                          n249 = case shown="True" w628 {
                            tunnel: w640 -> [w646 w650]
                            tunnel: [w646 w649] -> w620
                            tunnel: [0.0 ("Ampl Out") w648] -> w638
                            tunnel: w634 -> [_ w647]
                            frame False {
                            }
                            frame True {
                              n250 = local read "Flat_Cable_Data"() -> (w651:dbl[][])
                              n251 = call "GetCalData.vi"("Ary In"=w651, "error in (no error)"=w650, "RF Freq (MHz)"=w647) -> ("error out"=w649:errorcluster, "Ampl Out"=w648:dbl)  [unwired: 3 in, 4 out]
                            }
                          }
                          n252 = local read "SG1 delay(ms)"() -> (w639:i64)
                          n253 = local read "Sig Gen"() -> (w616:refnum<visa-resource-name>)
                          n254 = local read "Flatten Power to Set (dBm)"() -> (w637:dbl)
                          n255 = local read "Ary size(s)"() -> (w606:i32)
                          n256 = call "VSG_SET-GET_CW_1.00.vi"("Set Delay after (ms)"=w639, "Freq Units"="MHz", "error in"=w620, "Set Freq (MHz) num"=w634, "Session In"=w616) -> ("error out"=w619:errorcluster, "Session Out"=w617:refnum<visa-resource-name>)  [unwired: 3 in, 2 out]
                          n257 = local read "USB Power Meter"() -> (w627:refnum<visa-resource-name>)
                          n258 = Increment(x=w641) -> (x+1=w607:i32)
                          n259 = Divide(x=w607, y=w606) -> (x/y=w614:dbl)
                          n260 = Equal?(x=w607, y=w606) -> (x = y?=w622:bool)
                          n261 = call "SIGGEN_AMPL.vi"("Session In"=w617, "OFFS_IN"=w638, "Set Power (num)"=w637, "error in"=w619, "delay after set (ms)"=w639) -> ("error out"=w618:errorcluster)  [unwired: 7 in, 3 out]
                          n262 = local read "stop"() -> (w621:bool)
                          n263 = call "Configure Correction Frequency.vi"("error in (no error)"=w618, "Frequency (5E+7 Hz)"=w631, "VISA resource name"=w627) -> ("error out"=w636:errorcluster, "VISA resource name out"=w629:refnum<visa-resource-name>)  [unwired: 7 in]
                          n264 = Multiply(x=w614, y=100.0) -> (x*y=w611:dbl)
                          n265 = Or(x=w621, y=w622) -> (x .or. y?=w644:bool)
                          n266 = call "Read Measurement.vi"("error in (no error)"=w636, "VISA resource name"=w629) -> ("error out"=w633:errorcluster, "Measurement"=w635:dbl)  [unwired: 7 in, 1 out]
                          n267 = Number To Decimal String(number=w611) -> (decimal integer string=w612:string)  [unwired: 1 in]
                          n268 = local read "sg_flat_temp"() -> (w626:path)
                          n269 = Concatenate Strings("Input Cal " ("string"), w612, "% Complete" ("Label.Text")) -> (w613:string)
                          n270 = Build Array(w634, w635) -> (w632:dbl[])
                          n271 = local write "Power Meter"(w632) -> ()
                          n272 = control-ref of="Progress"() -> (w615:refnum<vi>)
                          n273 = property class="Slide (strict)"(reference=w615, "Caption.Text"=w613, "Value"=w611) -> ()  [unwired: 1 in, 2 out]
                          n274 = call-poly <vilib>:"Write Delimited Spreadsheet.vi"("file path (dialog if empty)"=w626, "1D data"=w632, "append to file? (new file:F)"=TRUE, "error in (no error)"=w633, "delimiter (\\t)"="," ("delimiter (\\t)")) -> ("error out"=w624:errorcluster)  [unwired: 9 in, 1 out]
                          n275 = Or(x=w644, y=w624) -> (x .or. y?=w625:bool)
                        }
                        n276 = local read "Sig Gen"() -> (w593:refnum<visa-resource-name>)
                        n277 = call "VSG_SET_RF_STATE_1.00.vi"("RF ON/OFF (OFF)"=FALSE, "error in"=w584, "Session In"=w593) -> ("error out"=w591:errorcluster, "Session Out"=w590:refnum<visa-resource-name>)  [unwired: 6 in, 1 out]
                        n278 = call "VISA_LCL.vi"("error in"=w591, "Session In"=w590) -> ("error out"=w605:errorcluster)  [unwired: 8 in, 1 out]
                        n279 = Select(t="FLAT Cal Complete!!!", s=w603, f="FLAT Cal NOT Complete!!!") -> (s? t:f=w580:string)
                      }
                      frame #3 {
                        n280 = call "ATE-CalPopup.vi"("Enable"=w655, "Message"=w654) -> ("OK"=w653:bool)  [unwired: 8 in, 1 out]
                        n281 = Not(x=w653) -> (.not. x?=w652:bool)
                      }
                    }
                  }
                }
              }
              frame 2 {
                n282 = property on="Path" class="Ring (strict)"() -> ("Strings []"=w673:string[])  [unwired: 2 in, 2 out]
                n283 = Index Array(array=w673, index=w672) -> (element=→"Path_out(str)":string)
                n284 = flat-sequence {
                  tunnel: w668 -> [w676]
                  tunnel: [w677] -> w658
                  tunnel: w658 -> [w684]
                  tunnel: [w683] -> w657
                  tunnel: [w695] -> w667
                  tunnel: w657 -> [w695]
                  tunnel: [w703] -> w669
                  tunnel: w667 -> [w704]
                  tunnel: [w717] -> w670
                  tunnel: w669 -> [w719]
                  tunnel: w670 -> [w733]
                  tunnel: [w732] -> w665
                  tunnel: [w731] -> w663
                  tunnel: [w730] -> w662
                  tunnel: w665 -> [w791]
                  tunnel: [w792] -> w664
                  tunnel: w663 -> [w790]
                  tunnel: w662 -> [w789]
                  tunnel: [w788] -> w661
                  tunnel: [w787] -> w659
                  tunnel: w664 -> [w803]
                  tunnel: [w802] -> w666
                  tunnel: ["Calibration Complete !!!"] -> w660
                  tunnel: w659 -> [_]
                  frame #0 {
                    n285 = call "ATE-CalPopup.vi"("error in (no error)"=w676, "Enable"=TRUE, "Message"="Remove the Power Sensor from the Test Cable\nConnect the Test Cable to the Antenna Cable\nUse a quality 2.92mm Bullet(Thru)") -> ("error out"=w677:errorcluster)  [unwired: 7 in, 1 out]
                  }
                  frame #1 {
                    n286 = local read "Switch"() -> (w685:refnum<visa-resource-name>)
                    n287 = call "RfSwitch_WAM_ATE.vi"("VISA_IN"=w685, "error in"=w684, "Source"=enum16{"RFSM", "PNA"}."PNA", "T/R"=enum16{"TX", "RX"}."TX") -> ("error out"=w683:errorcluster)  [unwired: 10 in, 1 out]
                    n288 = local read "Status"() -> (w678:string)
                    n289 = call "BuildStrings_Return.vi"("Input String"=w678, "New String"="Setting The RF Switch for TX...") -> ("concatenated string"=w679:string)  [unwired: 7 in, 2 out]
                    n290 = local write "Status"(w679) -> ()
                  }
                  frame #2 {
                    n291 = local read "sg_flat_file"() -> (w689:path)
                    n292 = Not(x="Browse for Flatness File(t)") -> (.not. x?=w686:bool)
                    n293 = And(x=w686, y="Use Flatten File(t)") -> (x .and. y?=w688:bool)
                    n294 = case shown="True" w688 {
                      tunnel: w689 -> [_ w697]
                      tunnel: [dbl[][] [] ("array out") w699] -> w691
                      frame False {
                      }
                      frame True {
                        n295 = call "GetCalData.vi"("Open new file T"=TRUE, "cal file path (dialog if empty)"=w697) -> ("array out"=w699:dbl[][])  [unwired: 4 in, 5 out]
                      }
                    }
                    "Flat_Cable_Data" <- w691
                    n296 = local read "Status"() -> (w694:string)
                    n297 = call "BuildStrings_Return.vi"("Input String"=w694, "New String"="Running OUTPUT Calibration...") -> ("concatenated string"=w693:string)  [unwired: 7 in, 2 out]
                    n298 = local write "Status"(w693) -> ()
                  }
                  frame #3 {
                    w706 = 10000.0  # SET CF (MHz)
                    n299 = local read "SA_REF_LVL (dBm)"() -> (w709:string)
                    n300 = local read "SA_AVGs"() -> (w708:i16)
                    n301 = local read "SA"() -> (w707:refnum<visa-resource-name>)
                    n302 = local read "IsPSA?(t)"() -> (w700:bool)
                    n303 = call "SetupSpectrumAnalyzerForCal.vi"("VISA Refnum in"=w707, "Select INST"="INST SA", "IsPSA(t)"=w700, "RBW"="RBW(Hz)", "RefLvl"=w709, "ATT"="ATT", "AVG Count"=w708, "Internal Preamp (0: Off)"="Internal Preamp (0: Off)", "error in (no error)"=w704, "SET CF (MHz)"=w706, "Span(MHz)"="Span(MHz)") -> ("error out"=w703:errorcluster)  [unwired: 3 in, 1 out]
                  }
                  frame #4 {
                    w716 = u16 1 items=["Hz", "MHz", "GHz"] ("Units")
                    w723 = 1000.0  # Delay Time (ms)
                    n304 = local read "Browse for Flatness File(t)"() -> (w712:bool)
                    n305 = local read "sg_flat_temp"() -> (w714:path)
                    n306 = local read "Sig Gen"() -> (w725:refnum<visa-resource-name>)
                    n307 = Select(t="Flatness File(browse)", s=w712, f=w714) -> (s? t:f=w715:path)
                    n308 = call "Visa_Reset_Clear.vi"("VISA resource name"=w725, "Send *CLS"=TRUE, "Restore Defaults"=TRUE, "Close VISA session"=FALSE, "error in (no error)"=w719, "Send *RST"=TRUE) -> ("VISA resource name Out"=w729:refnum<visa-resource-name>, "error out"=w726:errorcluster)  [unwired: 8 in]
                    n309 = call "UserFlatness.vi"("Units"=w716, "cal file path (dialog if empty)"=w715, "error in (no error)"=w726, "Session In"=w729) -> ("error out"=w727:errorcluster, "Session Out"=w728:refnum<visa-resource-name>)  [unwired: 5 in, 1 out]
                    n310 = call "VSG_SET_RF_STATE_1.00.vi"("RF ON/OFF (OFF)"=TRUE, "Delay Time (ms)"=w723, "error in"=w727, "Session In"=w728) -> ("error out"=w717:errorcluster)  [unwired: 5 in, 2 out]
                  }
                  frame #5 {
                    n311 = local read "Freq_MHz (ary)"() -> (w734:dbl[])
                    n312 = while {
                      tunnel: [w751] -> w732
                      tunnel: w734 -> [w760] mode=indexing
                      tunnel: w733 -> [w774]
                      tunnel: [w746] -> w731
                      tunnel: [w747] -> w730
                      i -> [w775]
                      stop <- w752 stop-if-true
                      w764 = TRUE  # Use PK Search (T)
                      w765 = 20.0  # Max Power
                      n313 = case shown="True" FALSE {
                        tunnel: w774 -> [w779 w785]
                        tunnel: [w779 w784] -> w773
                        tunnel: [0.0 ("Ampl Out") w783] -> w770
                        tunnel: w760 -> [_ w782]
                        frame False {
                        }
                        frame True {
                          n314 = local read "Flat_Cable_Data"() -> (w786:dbl[][])
                          n315 = call "GetCalData.vi"("Open new file T"=FALSE, "Ary In"=w786, "error in (no error)"=w785, "RF Freq (MHz)"=w782) -> ("error out"=w784:errorcluster, "Ampl Out"=w783:dbl)  [unwired: 2 in, 4 out]
                        }
                      }
                      n316 = local read "Output Power to Set (dBm)"() -> (w762:dbl)
                      n317 = local read "SG1 delay(ms)"() -> (w771:i64)
                      n318 = local read "IsPSA?(t)"() -> (w735:bool)
                      n319 = local read "Sig Gen"() -> (w754:refnum<visa-resource-name>)
                      n320 = call "SIGGEN_AMPL.vi"("Session In"=w754, "Max Power"=w765, "OFFS_IN"=w770, "Set Power (num)"=w762, "error in"=w773, "delay after set (ms)"=w771) -> ("Session Out"=w769:refnum<visa-resource-name>, "error out"=w772:errorcluster)  [unwired: 6 in, 2 out]
                      n321 = local read "Ary size(s)"() -> (w736:i32)
                      n322 = call "VSG_SET-GET_CW_1.00.vi"("Set Delay after (ms)"=w771, "error in"=w772, "Set Freq (MHz) num"=w760, "Session In"=w769) -> ("error out"=w768:errorcluster)  [unwired: 4 in, 3 out]
                      n323 = Increment(x=w775) -> (x+1=w737:i32)
                      n324 = local read "SA"() -> (w753:refnum<visa-resource-name>)
                      n325 = Divide(x=w737, y=w736) -> (x/y=w744:dbl)
                      n326 = call "SpecAnMeasCW_Cal.vi"("VISA Refnum in"=w753, "IsPSA(t)"=w735, "Use PK Search (T)"=w764, "SET CF (MHz) in"=w760, "error in (no error)"=w768) -> ("Ampl"=w759:dbl, "error out"=w767:errorcluster)  [unwired: 6 in, 3 out]
                      n327 = Multiply(x=w744, y=100.0) -> (x*y=w741:dbl)
                      n328 = Subtract(x=w759, y=w762) -> (x-y=w761:dbl)
                      n329 = Build Array(w760, w759) -> (→"Spec An":dbl[])
                      n330 = Number To Decimal String(number=w741) -> (decimal integer string=w742:string)  [unwired: 1 in]
                      n331 = local read "out_cal_tmp"() -> (w750:path)
                      n332 = Concatenate Strings("Input Cal " ("string"), w742, "% Complete" ("Label.Text")) -> (w743:string)
                      n333 = Equal?(x=w737, y=w736) -> (x = y?=w746:bool)
                      n334 = Build Array(w760, w761) -> (w757:dbl[])
                      n335 = control-ref of="Progress"() -> (w745:refnum<vi>)
                      n336 = local read "stop"() -> (w766:bool)
                      n337 = Index Array(array=w757, index=1) -> (element=→"SA_Offset":dbl)
                      n338 = property class="Slide (strict)"(reference=w745, "Caption.Text"=w743, "Value"=w741) -> ()  [unwired: 1 in, 2 out]
                      n339 = Or(x=w766, y=w746) -> (x .or. y?=w778:bool)
                      n340 = call-poly <vilib>:"Write Delimited Spreadsheet.vi"("file path (dialog if empty)"=w750, "1D data"=w757, "append to file? (new file:F)"=TRUE, "error in (no error)"=w767, "delimiter (\\t)"="," ("delimiter (\\t)")) -> ("error out"=w751:errorcluster)  [unwired: 9 in, 1 out]
                      n341 = Or(x=w778, y=w751) -> (x .or. y?=w752:bool)
                      n342 = Select(t="OUTPUT Cal Complete!!", s=w746, f="OUTPUT Cal Error!!") -> (s? t:f=w747:string)
                    }
                  }
                  frame #6 {
                    n343 = case shown="True" w790 {
                      selector: w790 -> [_ w798]
                      tunnel: [w795 w800] -> w792
                      tunnel: w791 -> [w795 w799]
                      tunnel: w789 -> [w793 w797]
                      tunnel: [TRUE ("OK") w796] -> w788
                      tunnel: [w793 w797] -> w787
                      frame False {
                      }
                      frame True {
                        n344 = call "ATE-CalPopup.vi"("error in (no error)"=w799, "Enable"=w798, "Message"=w797) -> ("error out"=w800:errorcluster, "OK"=w796:bool)  [unwired: 7 in]
                      }
                    }
                  }
                  frame #7 {
                    n345 = local read "Sig Gen"() -> (w807:refnum<visa-resource-name>)
                    n346 = call "VSG_SET_RF_STATE_1.00.vi"("RF ON/OFF (OFF)"=FALSE, "error in"=w803, "Session In"=w807) -> ("error out"=w805:errorcluster, "Session Out"=w808:refnum<visa-resource-name>)  [unwired: 6 in, 1 out]
                    n347 = call "VISA_LCL.vi"("error in"=w805, "Session In"=w808) -> ("error out"=w806:errorcluster)  [unwired: 8 in, 1 out]
                    n348 = local read "SA"() -> (w809:refnum<visa-resource-name>)
                    n349 = call "VISA_LCL.vi"("error in"=w806, "Session In"=w809) -> ("error out"=w802:errorcluster)  [unwired: 8 in, 1 out]
                  }
                }
              }
              frame 3 {
              }
            }
            n350 = local read "Select AutoCal(T)"() -> (w325:bool)
            n351 = Not(x=w325) -> (.not. x?=w324:bool)
            n352 = Or(x=w329, y=w324) -> (x .or. y?=w326:bool)
          }
        }
        frame True {
        }
      }
      n353 = case shown="False" w309 {
        tunnel: w313 -> [w818 w822]
        tunnel: w311 -> [w816 w821]
        tunnel: [w818 w820] -> w310
        tunnel: [FALSE ("OK") w819] -> w308
        frame False {
          n354 = call "Display Message to User6"("Message"=w816) -> ()  [unwired: 9 in, 2 out]
        }
        frame True {
          n355 = call "Display Message to User4"("error in (no error)"=w822, "Message"=w821) -> ("error out"=w820:errorcluster, "OK"=w819:bool)  [unwired: 8 in]
        }
      }
      n356 = local write "OK(t)"(w308) -> ()
    }
    frame #6 {
      n357 = local read "OK(t)"() -> (w825:bool)
      n358 = case shown="True" w825 {
        tunnel: w824 -> [w826 w827]
        tunnel: [w826 w827] -> w823
        frame False {
        }
        frame True {
          n359 = local read "sg_flat_temp"() -> (w836:path)
          n360 = local read "out_cal_tmp"() -> (w837:path)
          n361 = local read "in_cal_temp"() -> (w838:path)
          n362 = local read "out_cal_file"() -> (w834:path)
          n363 = local read "sg_flat_file"() -> (w833:path)
          n364 = local read "in_cal_file"() -> (w835:path)
          n365 = Build Array(w838, w837, w836) -> (w831:path[])
          n366 = Build Array(w835, w834, w833) -> (w830:path[])
          n367 = Build Array(w831, w830) -> (w832:path[][])
          n368 = Array Size(array=w830) -> (size(s)=w829:i32)
          n369 = Transpose 2D Array(2D array=w832) -> (transposed array=w828:path[][])
          n370 = while {
            tunnel: w828 -> [w851] mode=indexing
            tunnel: w829 -> [w842]
            i -> [w840]
            stop <- w841 stop-if-true
            n371 = Index Array(array=w851) -> (element #1=w846:path, element #2=w843:path)  [unwired: 2 in]
            n372 = Increment(x=w840) -> (x+1=w839:i32)
            n373 = Path To String(path=w846) -> (string=w847:string)
            n374 = Path To String(path=w843) -> (string=w844:string)
            n375 = Equal?(x=w842, y=w839) -> (x = y?=w841:bool)
            n376 = Concatenate Strings("Do You Want to Move the Cal File : " ("string"), w847, " to " ("string"), w844) -> (w848:string)
            n377 = call "Display Message to User5"("Message"=w848) -> ("SAVE FILE"=w850:bool)  [unwired: 9 in, 1 out]
            n378 = case shown="False" w850 {
              tunnel: w846 -> [w853 w855]
              tunnel: w843 -> [_ w854]
              frame False {
                n379 = Delete(path (use dialog)=w853, confirm (F)=FALSE) -> ()  [unwired: 3 in, 3 out]
              }
              frame True {
                n380 = Move(source path=w855, 10:w854) -> ()  [unwired: 3 in, 3 out]
              }
            }
          }
        }
      }
    }
    frame #7 {
      n381 = disable-structure shown="Disabled" {
        frame Disabled {
          n382 = property class="VI"() -> (reference out=w860:refnum<vi>, "FP.State"=w858:T2)  [unwired: 2 in, 1 out]
          n383 = Equal?(x=w858, y=T2."Closed") -> (x = y?=w859:bool)
          n384 = case shown="True" w859 {
            tunnel: w860 -> [w862 _]
            frame False {
              n385 = invoke class="VI" method="FP.Close"(reference=w862) -> (reference out=w861:refnum<vi>)  [unwired: 2 in, 2 out]
              n386 = invoke class="VI" method="Abort VI"(reference=w861) -> ()  [unwired: 2 in, 3 out]
            }
            frame True {
              n387 = invoke class="VI" method="Abort VI"() -> ()  [unwired: 3 in, 3 out]
            }
          }
        }
        frame Enabled {
        }
      }
      "error out" <- w856
    }
  }
